vi "acquisition-main.vi"(7 "acquisition-input-cluster":T4={"detector"=0, "HBinning"=1, "readout mode"=0, "ready"=FALSE, "Exposure Time Read"=0.0, "select background"=enum."single", "xeva-camref"=refnum} {"Exposure Time Read" format="%.2g"; "readout mode" items=["Full Vertical Binning", "Image", "Vertical Binning"]; "HBinning" items=["1x"=1, "2x"=2, "4x"=4, "8x"=8, "16x"=16]; "detector" items=["Newton", "iDus", "Clara", "Xeva"]}, 8 "error in":errorcluster, 9 "Progress In":T2 {"Progress" scale=0.0..100.0}, 10 "Data In":cluster{"Measurement":i32[], "Background":i32[]}, 11 "input action":T1(ring)) -> (0 "error out":errorcluster, 1 "Progress Out":T2 {"Progress" scale=0.0..100.0}, 2 "Data Out":cluster{"Measurement":i32[], "Background":i32[]}, 3 "next action":T1(ring))   [LabVIEW 2017]
uses:
  <vilib>/Xenics Infrared Solutions/Xeneth LabVIEW API/VIs/Controls/Camara.ctl
  <vilib>/Xenics Infrared Solutions/Xeneth LabVIEW API/Xeneth.lvlib
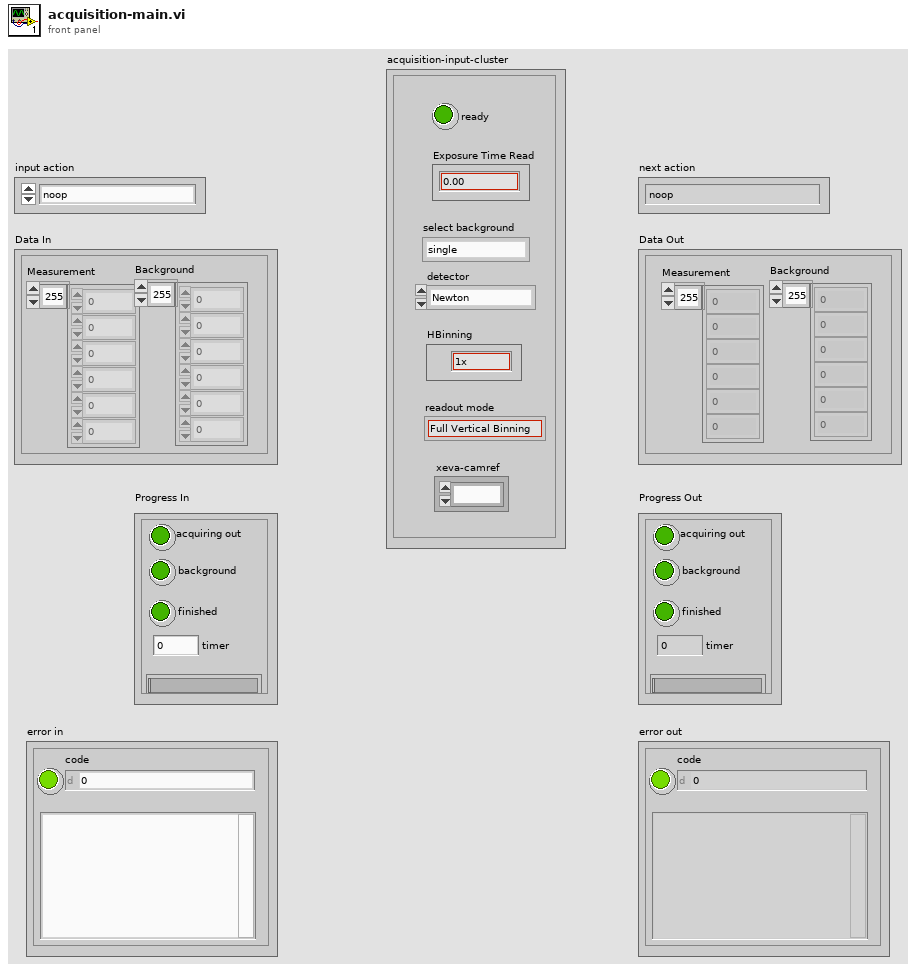
[diagram p1: front panel]
types:
  T1 = enum16{"noop", "set background", "set measurement", "start acquisition", "abort", "get Data", "check progress", "restart acquisition", "start", "acquisition finished", "measurement finished", "wait to continue", "wait for ready"}
  T2 = cluster{"acquiring out":bool, "Progress":u8, "background":bool, "timer":u32, "finished":bool}
  T3 = typedef "Xeneth.lvlib/Camara.ctl" = refnum<k1>
  T4 = cluster{"detector":u16, "HBinning":u16, "readout mode":u16, "ready":bool, "Exposure Time Read":sgl, "select background":enum16{"skip", "single", "multiple"}, "xeva-camref":T3}
  T5 = cluster{"detector":u16, "HBinning":u16, "readout mode":u16}
  T6 = enum16{"noop", "set background", "set measurement", "start acquisition", "abort", "get Data", "check progress", "restart acquisition", "start", "acquisition finished", "measurement finished", "wait to continue"}
  T7 = enum16{"noop", "set background", "set measurement", "start acquisition", "abort acquisition", "get Data", "check progress", "restart measurement"}
  T8 = enum16{"noop", "set background", "set measurement", "start acquisition", "abort", "get Data", "check progress", "restart acquisition", "start", "acquisition finished", "start next measurement", "wait to continue"}
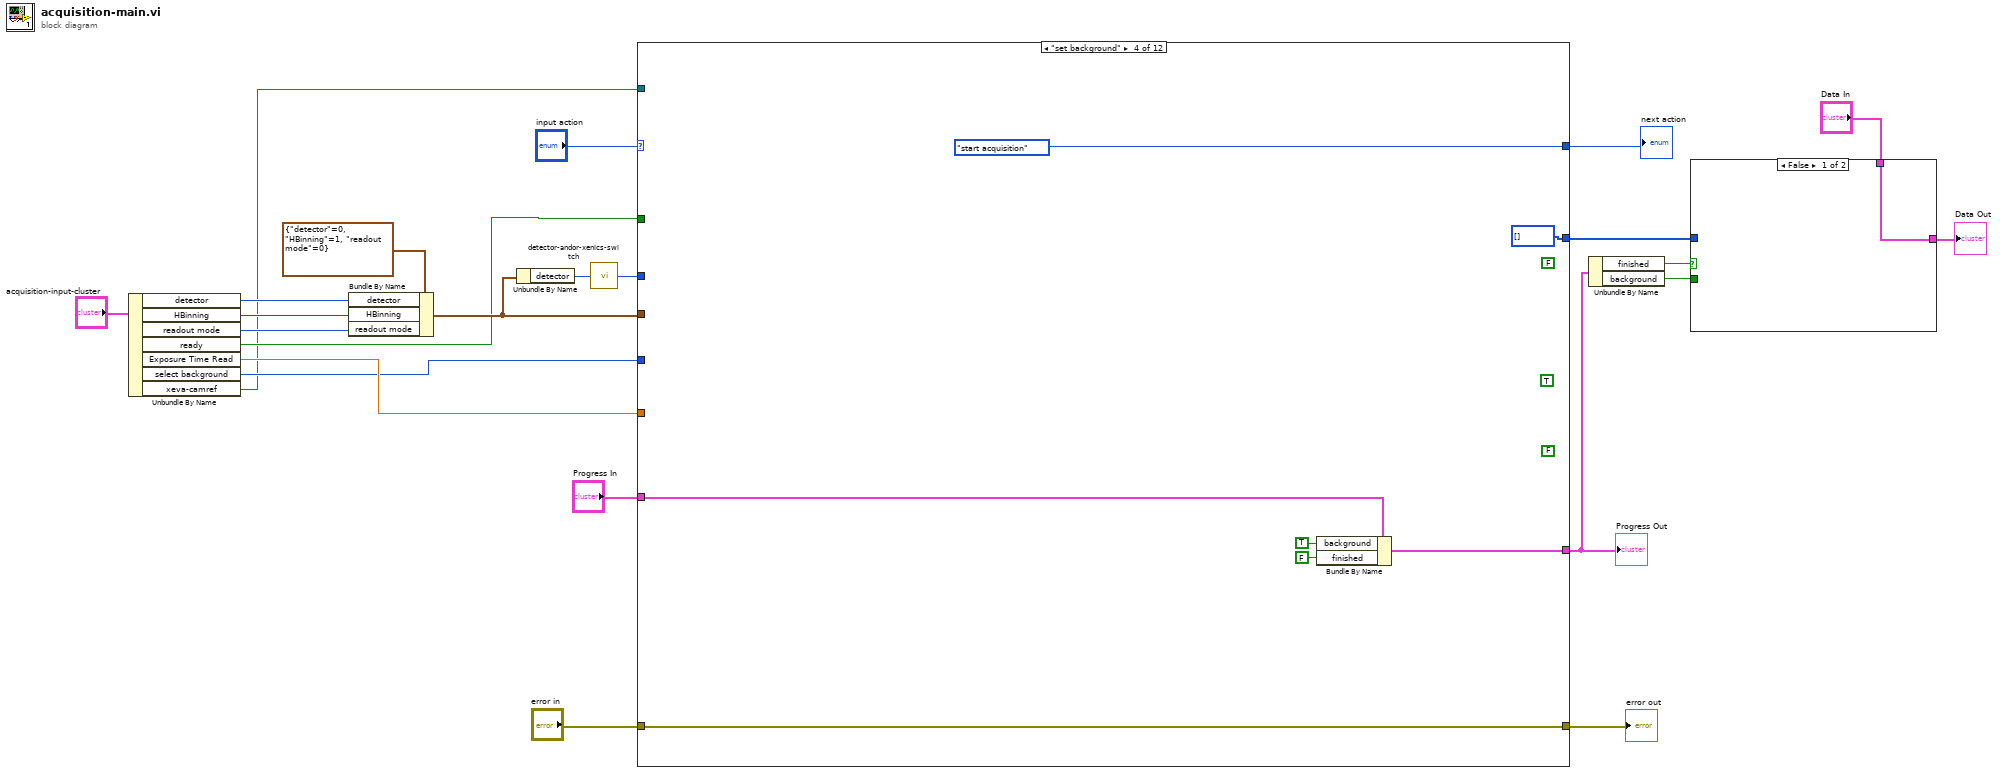
[diagram p0: block diagram]
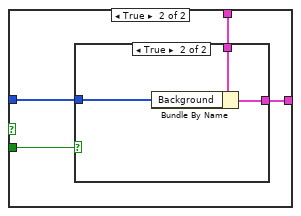
[diagram p2: hidden frame]
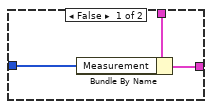
[diagram p3: hidden frame]
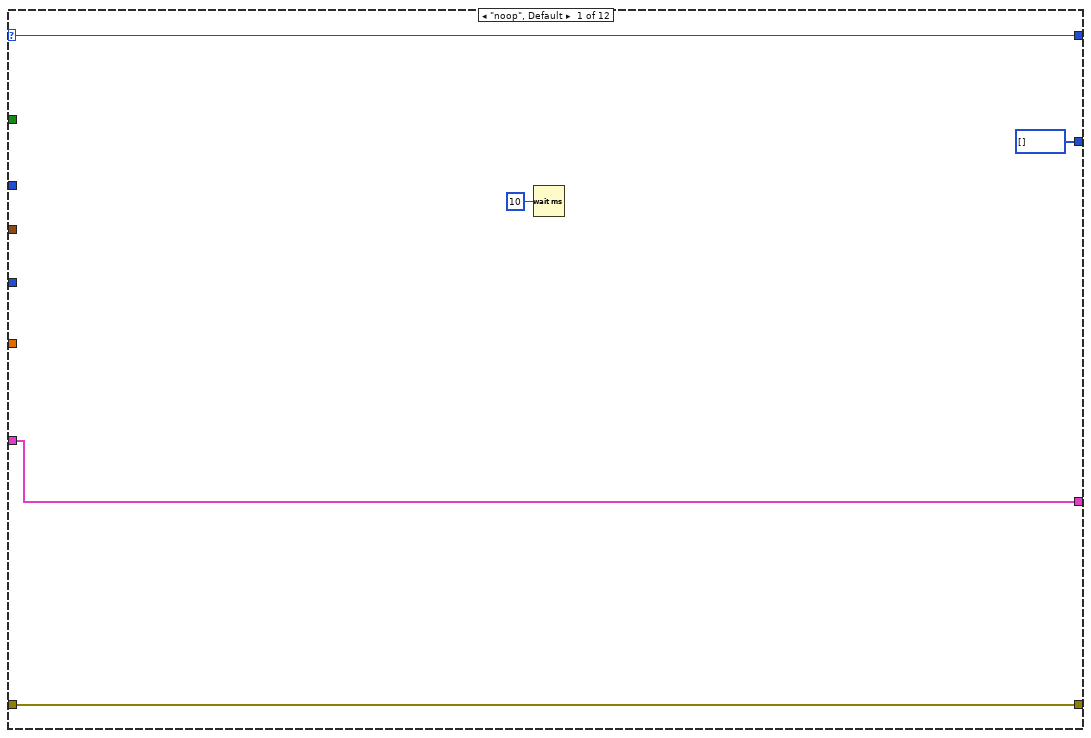
[diagram p4: hidden frame]
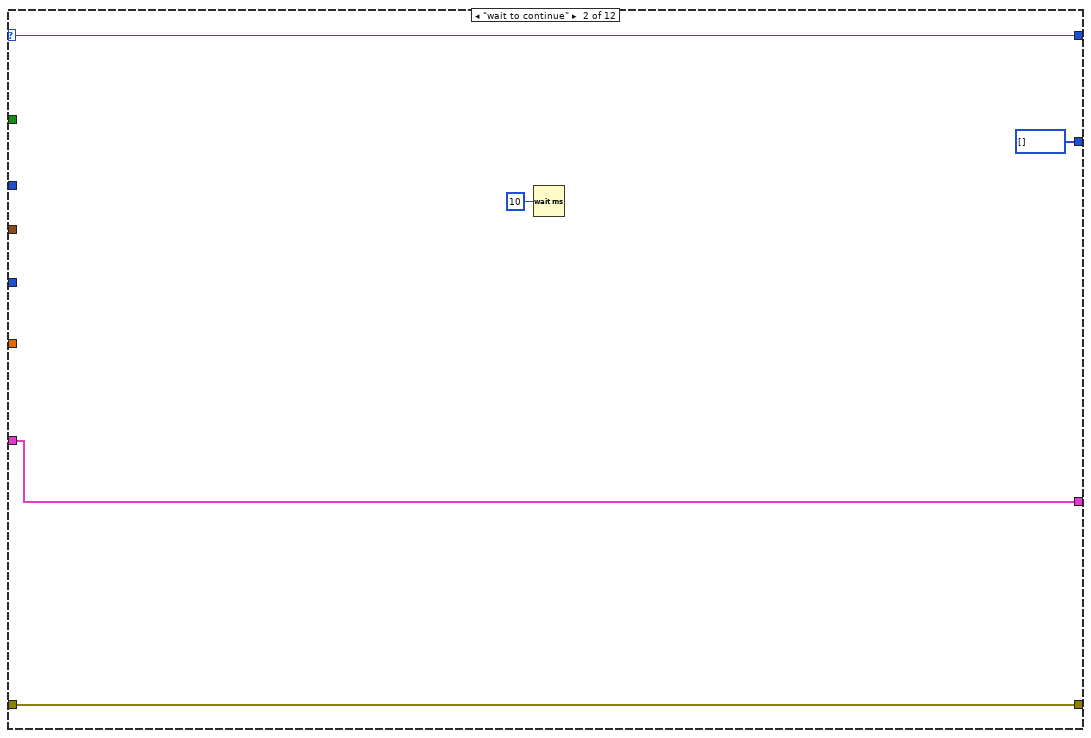
[diagram p5: hidden frame]
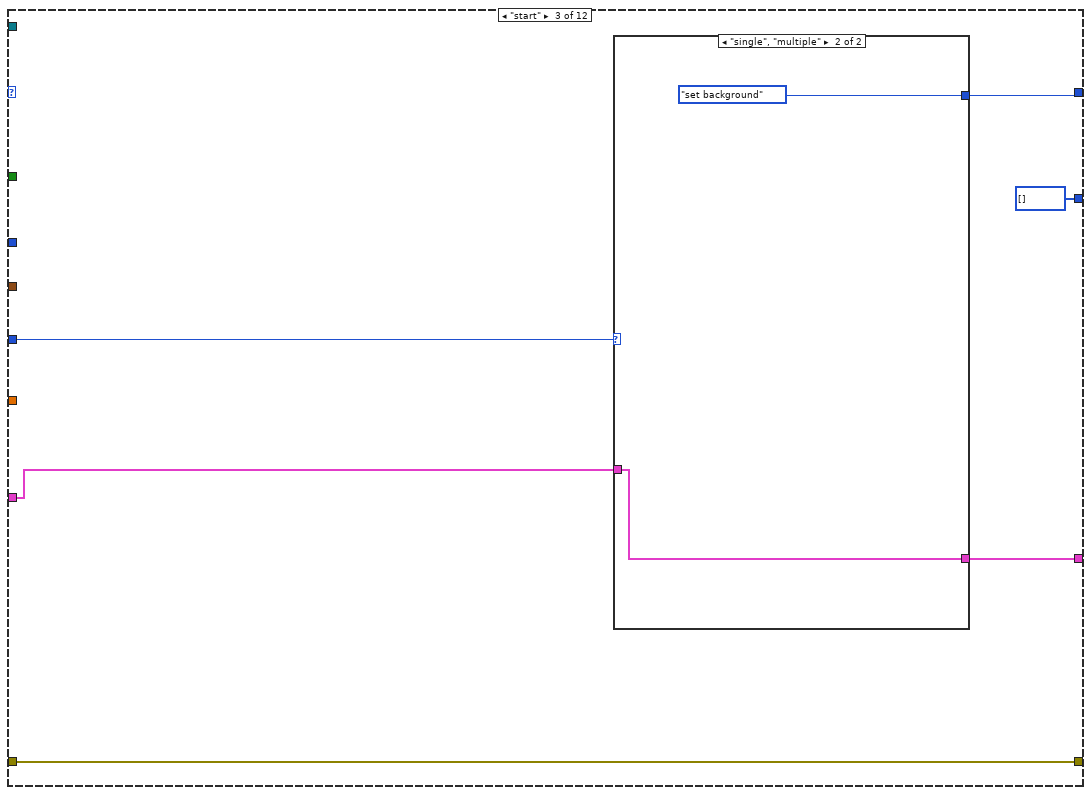
[diagram p6: hidden frame]
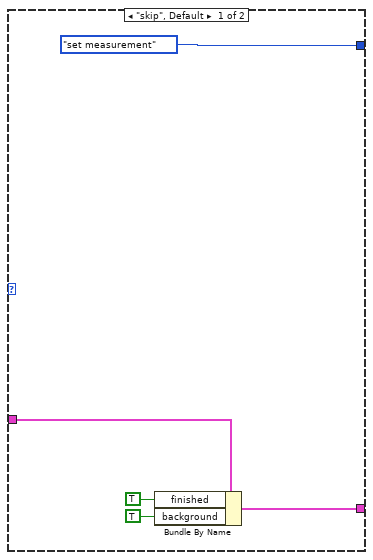
[diagram p7: hidden frame]
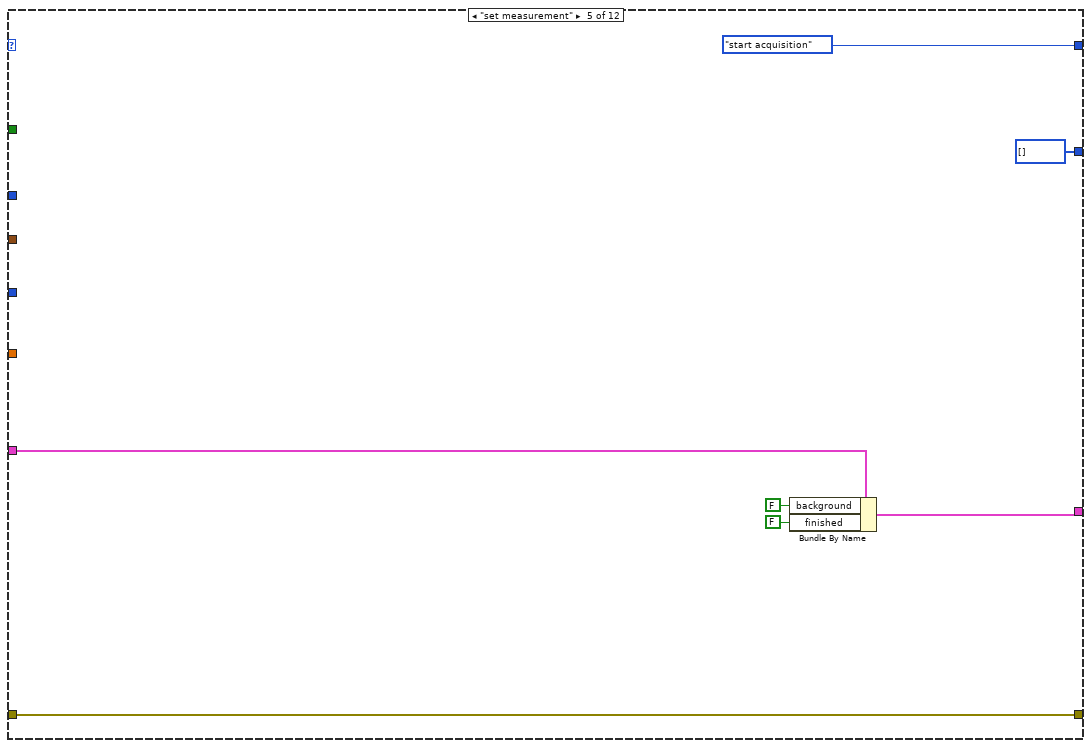
[diagram p8: hidden frame]
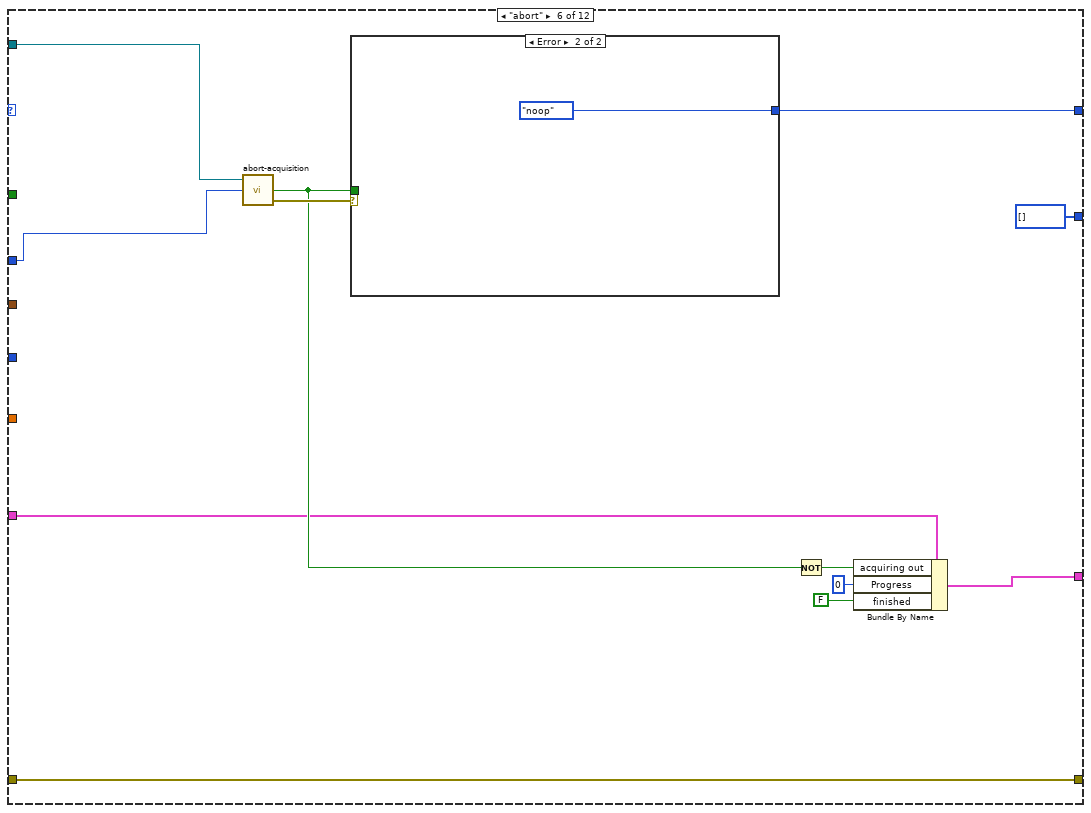
[diagram p9: hidden frame]
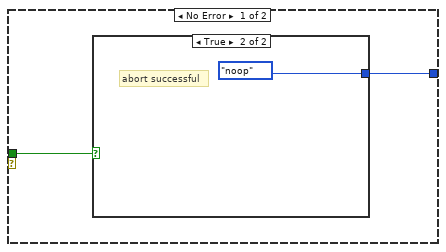
[diagram p10: hidden frame]
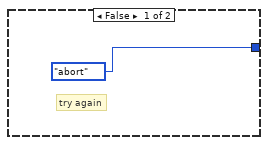
[diagram p11: hidden frame]
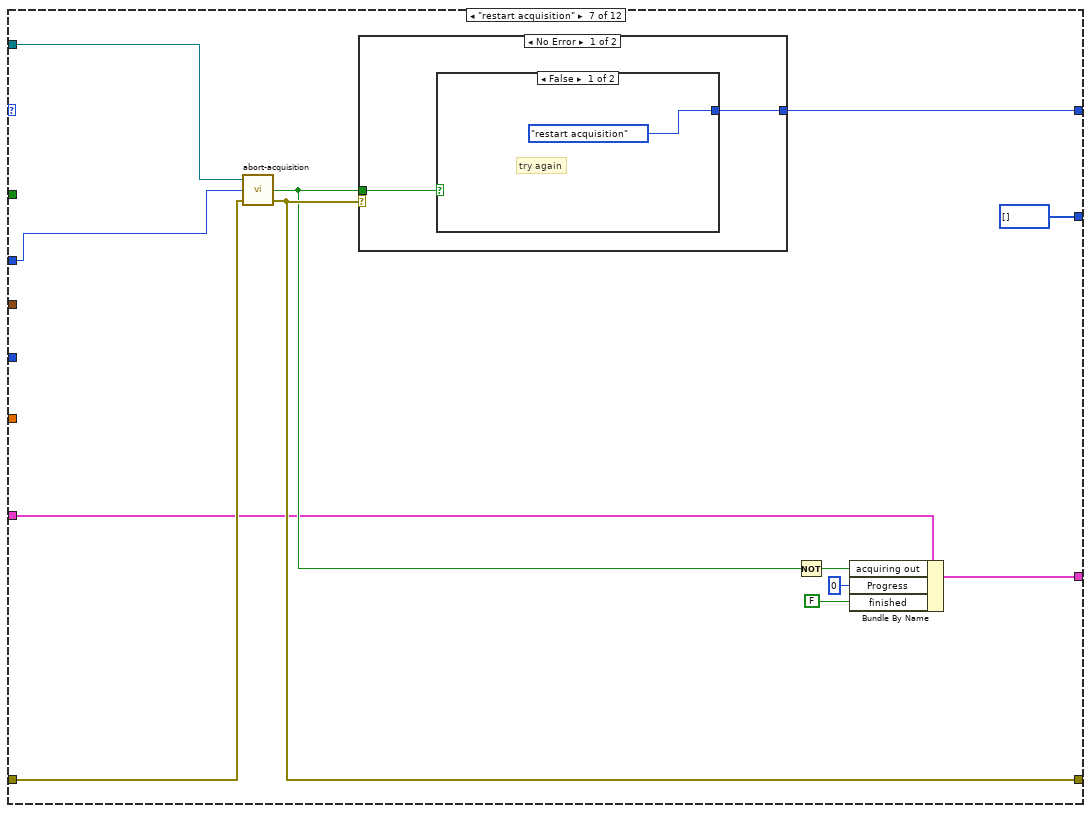
[diagram p12: hidden frame]
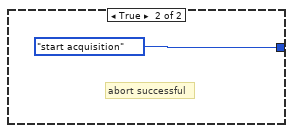
[diagram p13: hidden frame]
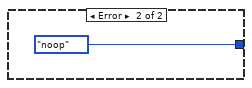
[diagram p14: hidden frame]
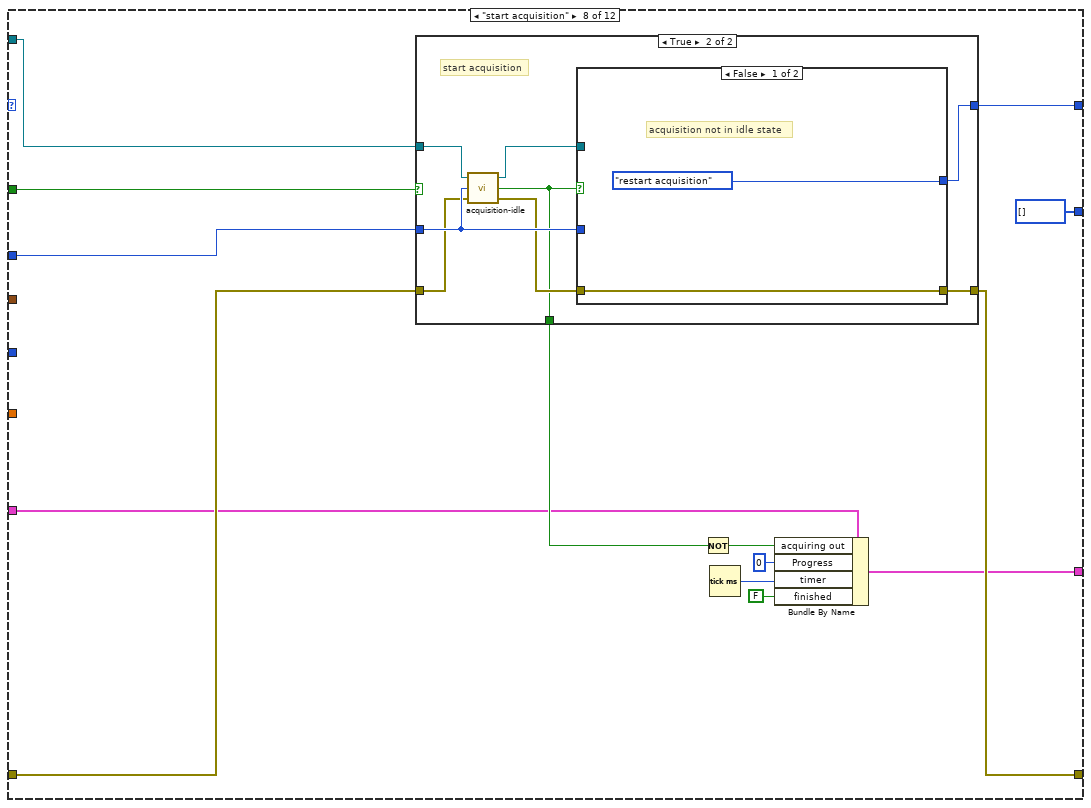
[diagram p15: hidden frame]
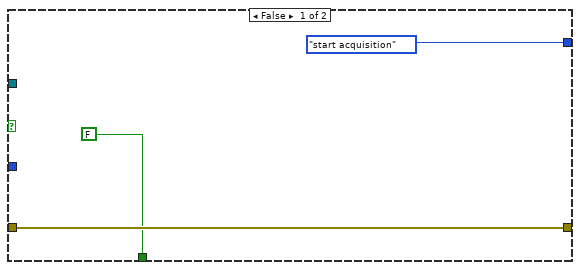
[diagram p16: hidden frame]
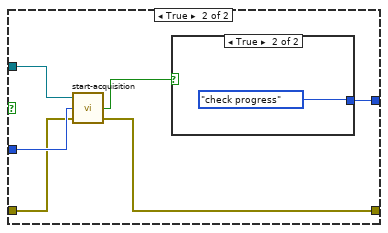
[diagram p17: hidden frame]
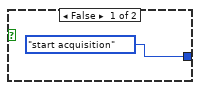
[diagram p18: hidden frame]
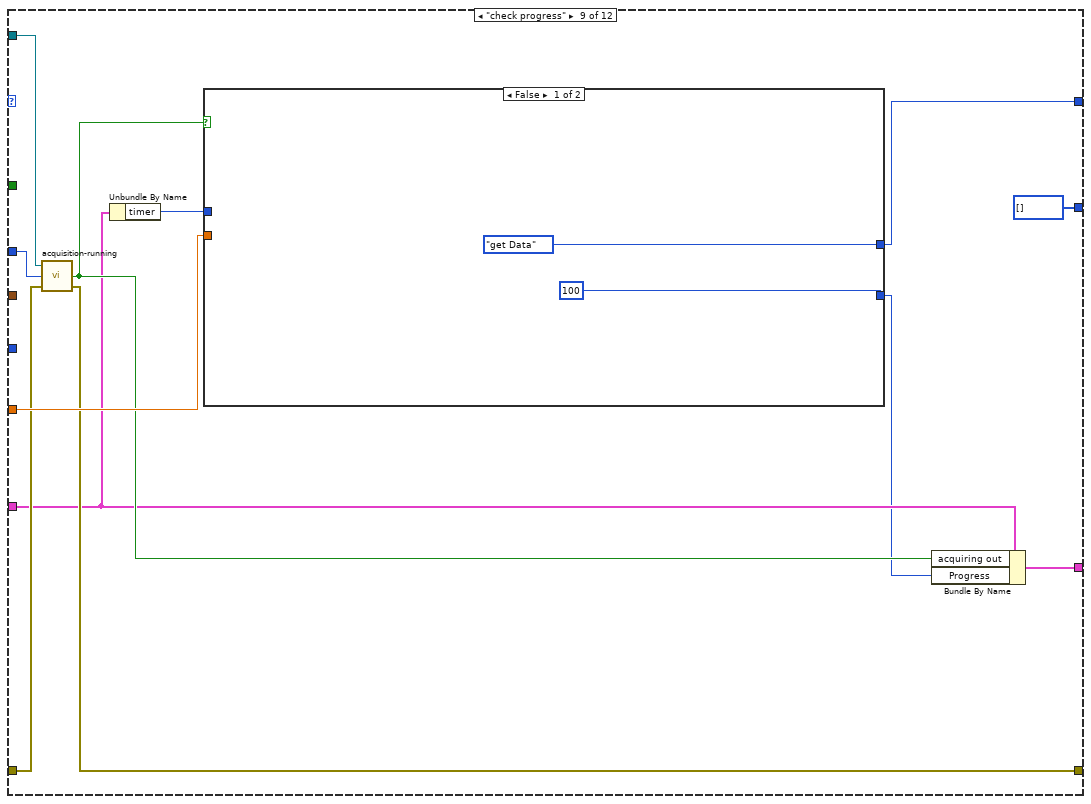
[diagram p19: hidden frame]
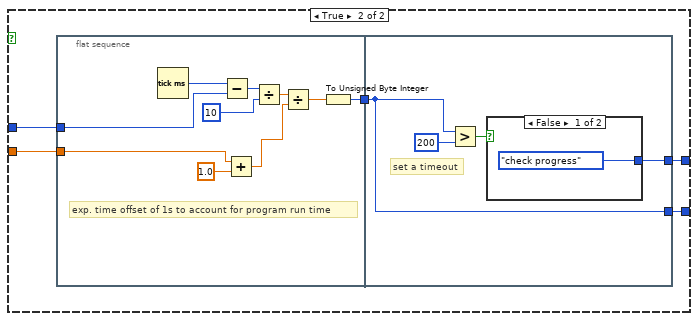
[diagram p20: hidden frame]
diagram:
  n1 = Unbundle By Name("acquisition-input-cluster") -> ("detector"=w16:u16, "HBinning"=w15:u16, "readout mode"=w14:u16, "ready"=w13:bool, "Exposure Time Read"=w12:sgl, "select background"=w11:enum16{"skip", "single", "multiple"}, "xeva-camref"=w10:T3)
  n2 = Bundle By Name(cluster=T5 {"detector"=0, "HBinning"=1, "readout mode"=0} ("andor-get-data-cluster"), "detector"=w16, "HBinning"=w15, "readout mode"=w14) -> (w18:T5)
  n3 = Unbundle By Name(w18) -> ("detector"=w22:u16)
  n4 = call "detector-andor-xenics-switch.vi"("Detector"=w22) -> ("Manufacturer"=w21:enum16{"Andor", "Xenics", "unknown"})
  n5 = case shown="\"set background\"" "input action" {
    selector: "input action" -> [w28 w33 _ _ _ _ _ _ _ _ _ _]
    tunnel: w10 -> [_ _ _ _ _ w71 w89 w108 w137 w173 _ _]
    tunnel: [w28 w33 w36 T6."start acquisition" ("next action") T6."start acquisition" ("next action") w70 w88 w107 w141 w166 w180 w192] -> w1
    tunnel: w13 -> [_ _ _ _ _ _ _ w106 _ _ _ _]
    tunnel: [w27 w32 w37 w53 w60 w68 w86 w105 w138 w167 w181 w190] -> w23
    tunnel: "error in" -> [w27 w32 w37 w53 w60 w68 w87 w104 w139 w175 w181 w190]
    tunnel: w12 -> [_ _ _ _ _ _ _ _ w140 _ _ _]
    tunnel: w21 -> [_ _ _ _ _ w69 w85 w103 w136 _ _ _]
    tunnel: w18 -> [_ _ _ _ _ _ _ _ _ w174 _ _]
    tunnel: [i32[] [] ("raw-data") i32[] [] ("raw-data") i32[] [] ("raw-data") i32[] [] ("raw-data") i32[] [] ("raw-data") i32[] [] ("raw-data") i32[] [] ("raw-data") i32[] [] ("raw-data") i32[] [] ("raw-data") w172 i32[] [] ("raw-data") i32[] [] ("raw-data")] -> w7
    tunnel: w11 -> [_ _ w39 _ _ _ _ _ _ _ _ w193]
    tunnel: "Progress In" -> [w25 w30 w35 w50 w55 w65 w79 w98 w132 w170 w185 w189]
    tunnel: [w25 w30 w34 w51 w56 w62 w81 w99 w133 w171 w184 w189] -> w5
    frame "noop", Default {
      n6 = Wait (ms)(milliseconds to wait=u32 10) -> ()  [unwired: 1 out]
    }
    frame "wait to continue" {
      n7 = Wait (ms)(milliseconds to wait=u32 10) -> ()  [unwired: 1 out]
    }
    frame "start" {
      n8 = case shown="\"single\", \"multiple\"" w39 {
        tunnel: [T6."set measurement" ("next action") T6."set background" ("next action")] -> w36
        tunnel: w35 -> [w42 w46]
        tunnel: [w41 w46] -> w34
        frame "skip", Default {
          n9 = Bundle By Name(cluster=w42, "finished"=TRUE, "background"=TRUE ("finished")) -> (w41:T2)
        }
        frame "single", "multiple" {
        }
      }
    }
    frame "set background" {
      (unwired) FALSE ("acquiring")
      (unwired) FALSE ("acquisition finished")
      (unwired) TRUE ("background")
      n10 = Bundle By Name(cluster=w50, "background"=TRUE, "finished"=FALSE) -> (w51:T2)
    }
    frame "set measurement" {
      n11 = Bundle By Name(cluster=w55, "background"=FALSE, "finished"=FALSE) -> (w56:T2)
    }
    frame "abort" {
      n12 = call "abort-acquisition.vi"("Manufacturer"=w69, "Cam Ref"=w71) -> ("error out"=w72:errorcluster, "aborted"=w66:bool)  [unwired: 1 in, 1 out]
      n13 = case shown="Error" w72 {
        tunnel: w66 -> [w74 _]
        tunnel: [w73 T6."noop" ("next action")] -> w70
        frame No Error {
          n14 = case shown="True" w74 {
            tunnel: [T6."abort" ("next action") T6."noop" ("next action")] -> w73
            frame False {
              # "try again"
            }
            frame True {
              # "abort successful"
            }
          }
        }
        frame Error {
        }
      }
      n15 = Not(x=w66) -> (.not. x?=w64:bool)
      n16 = Bundle By Name(cluster=w65, "acquiring out"=w64, "Progress"=u8 0, "finished"=FALSE) -> (w62:T2)
    }
    frame "restart acquisition" {
      n17 = call "abort-acquisition.vi"("error in (no error)"=w87, "Manufacturer"=w85, "Cam Ref"=w89) -> ("error out"=w86:errorcluster, "aborted"=w83:bool)  [unwired: 1 out]
      n18 = case shown="No Error" w86 {
        tunnel: w83 -> [w91 _]
        tunnel: [w90 T7."noop" ("input action")] -> w88
        frame No Error {
          n19 = case shown="False" w91 {
            tunnel: [T6."restart acquisition" ("next action") T6."start acquisition" ("next action")] -> w90
            frame False {
              # "try again"
            }
            frame True {
              # "abort successful"
            }
          }
        }
        frame Error {
        }
      }
      n20 = Not(x=w83) -> (.not. x?=w80:bool)
      n21 = Bundle By Name(cluster=w79, "acquiring out"=w80, "Progress"=u8 0, "finished"=FALSE) -> (w81:T2)
    }
    frame "start acquisition" {
      n22 = case shown="True" w106 {
        tunnel: w103 -> [_ w119]
        tunnel: w108 -> [_ w118]
        tunnel: [T6."start acquisition" ("next action") w115] -> w107
        tunnel: [w111 w114] -> w105
        tunnel: w104 -> [w111 w113]
        tunnel: [FALSE ("acquiring") w112] -> w101
        frame False {
        }
        frame True {
          # "start acquisition"
          n23 = call "acquisition-idle.vi"("error in (no error)"=w113, "Manufacturer"=w119, "xeva-camref-in"=w118) -> ("error out"=w116:errorcluster, "camera idle"=w112:bool, "xeva-camref-out"=w117:T3)
          n24 = case shown="False" w112 {
            tunnel: w119 -> [_ w127]
            tunnel: w117 -> [_ w126]
            tunnel: w116 -> [w121 w125]
            tunnel: [T6."restart acquisition" ("next action") w123] -> w115
            tunnel: [w121 w124] -> w114
            frame False {
              # "acquisition not in idle state"
            }
            frame True {
              n25 = call "start-acquisition.vi"("error in (no error)"=w125, "Manufacturer"=w127, "xeva-camref-in"=w126) -> ("error out"=w124:errorcluster, "acqusition started"=w122:bool)  [unwired: 1 out]
              n26 = case shown="True" w122 {
                tunnel: [T6."start acquisition" ("next action") T6."check progress" ("next action")] -> w123
                frame False {
                }
                frame True {
                }
              }
            }
          }
        }
      }
      n27 = Not(x=w101) -> (.not. x?=w97:bool)
      n28 = Tick Count (ms)() -> (millisecond timer value=w96:u32)
      n29 = Bundle By Name(cluster=w98, "acquiring out"=w97, "Progress"=u8 0, "timer"=w96, "finished"=FALSE ("acquisition finished")) -> (w99:T2)
    }
    frame "check progress" {
      n30 = call "acquisition-running.vi"("error in (no error)"=w139, "Manufacturer"=w136, "xeva-camref-in"=w137) -> ("error out"=w138:errorcluster, "acquiring"=w134:bool)  [unwired: 1 out]
      n31 = Unbundle By Name(w132) -> ("timer"=w131:u32)
      n32 = case shown="False" w134 {
        tunnel: [T6."get Data" ("next action") w148] -> w141
        tunnel: w140 -> [_ w147]
        tunnel: w131 -> [_ w146]
        tunnel: [u8 100 w145] -> w130
        frame False {
        }
        frame True {
          n33 = flat-sequence {
            tunnel: w147 -> [w151]
            tunnel: w146 -> [w150]
            tunnel: [w149] -> w144
            tunnel: [w162] -> w148
            tunnel: [w159] -> w145
            tunnel: w144 -> [w159]
            frame #0 {
              # "exp. time offset of 1s to account for program run time"
              n34 = Tick Count (ms)() -> (millisecond timer value=w158:u32)
              n35 = Subtract(x=w158, y=w150) -> (x-y=w156:u32)
              n36 = Add(x=w151, y=sgl 1.0) -> (x+y=w153:sgl)
              n37 = Divide(x=w156, y=u32 10 ("millisecond timer value")) -> (x/y=w155:dbl)
              n38 = Divide(x=w155, y=w153) -> (x/y=w154:dbl)
              n39 = To Unsigned Byte Integer(number=w154) -> (unsigned 8bit integer=w149:u8)
            }
            frame #1 {
              # "set a timeout"
              n40 = Greater?(x=w159, y=u8 200) -> (0:w160:bool)
              n41 = case shown="False" w160 {
                tunnel: [T6."check progress" ("next action") T6."restart acquisition" ("next action")] -> w162
                frame False {
                }
                frame True {
                }
              }
            }
          }
        }
      }
      n42 = Bundle By Name(cluster=w132, "acquiring out"=w134, "Progress"=w130) -> (w133:T2)
    }
    frame "get Data" {
      n43 = call "get-data.vi"("error in (no error)"=w175, "andor-get-data-cluster"=w174, "xeva-camref-in"=w173) -> ("error out"=w167:errorcluster, "raw-data"=w172:i32[])  [unwired: 1 out]
      n44 = case shown="No Error" w167 {
        tunnel: [T6."acquisition finished" ("next action") T6."restart acquisition" ("next action")] -> w166
        tunnel: [TRUE ("acquiring out") FALSE ("acquiring out")] -> w165
        frame No Error {
        }
        frame Error {
        }
      }
      n45 = Bundle By Name(cluster=w170, "finished"=w165, "acquiring out"=FALSE, "Progress"=u8 100) -> (w171:T2)
    }
    frame "acquisition finished" {
      n46 = Unbundle By Name(w185) -> ("background"=w186:bool)
      n47 = case shown="True" w186 {
        tunnel: [T8."start next measurement" ("next action") T6."set measurement" ("next action")] -> w180
        frame False {
        }
        frame True {
          # "go for signal acquisition"
        }
      }
      n48 = Bundle By Name(cluster=w185, "finished"=FALSE) -> (w184:T2)
    }
    frame "measurement finished" {
      # "automatic restart"
      n49 = case shown="\"multiple\"" w193 {
        tunnel: [T6."set measurement" ("next action") T6."set background" ("next action")] -> w192
        frame "skip", "single", Default {
          # "no further background"
        }
        frame "multiple" {
        }
      }
    }
  }
  "error out" <- w23
  "Progress Out" <- w5
  "next action" <- w1
  n50 = Unbundle By Name(w5) -> ("finished"=w4:bool, "background"=w3:bool)
  n51 = case shown="False" w4 {
    tunnel: "Data In" -> [w196 w200]
    tunnel: [w196 w199] -> w8
    tunnel: w3 -> [_ w198]
    tunnel: w7 -> [_ w197]
    frame False {
    }
    frame True {
      n52 = case shown="True" w198 {
        tunnel: w200 -> [w201 w206]
        tunnel: [w202 w205] -> w199
        tunnel: w197 -> [w203 w204]
        frame False {
          n53 = Bundle By Name(cluster=w201, "Measurement"=w203) -> (w202:cluster{"Measurement":i32[], "Background":i32[]})
        }
        frame True {
          n54 = Bundle By Name(cluster=w206, "Background"=w204) -> (w205:cluster{"Measurement":i32[], "Background":i32[]})
        }
      }
    }
  }
  "Data Out" <- w8
